vi "Calculate tf.vi"(7 "Open Interval? (T)":bool=TRUE, 11 "Waveform":T1) -> (3 "Tf Out":timestamp)   [LabVIEW 2020, in "WavBuf.lvclass"]
uses:
  WavBuf.lvclass
  Universal Controls/Waveform_Data.ctl
  <vilib>/Waveform/WDTOps.llb/WDT Get Final Time Value DBL.vi
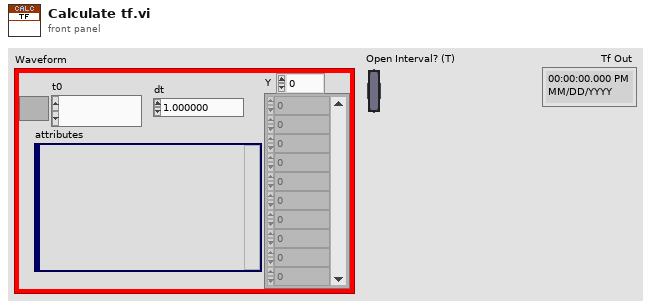
[diagram p1: front panel]
types:
  T1 = typedef "Waveform_Data.ctl" = waveform(dbl)
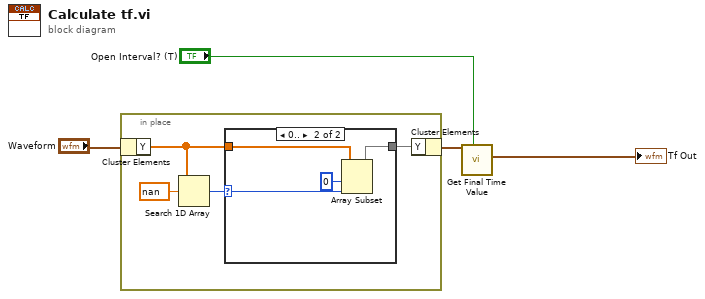
[diagram p0: block diagram]
diagram:
  n1 = in-place {
    n2 = in-place-cluster #1("Waveform") -> ("Y"=w6:dbl[])
    n3 = Search 1D Array(1D array=w6, element=nan) -> (index of element=w7:i32)  [unwired: 1 in]
    n4 = case shown="0.." w7 {
      selector: w7 -> [_ w10]
      tunnel: w6 -> [w9 w13]
      tunnel: [w9 w12] -> w5
      frame ..-1 {
      }
      frame 0.. {
        n5 = Array Subset(array=w13, index=0, length=w10) -> (w12:dbl[])
      }
    }
    n6 = in-place-cluster #1("Y"=w5) -> (w1:T1)
  }
  n7 = call-poly <vilib>:"Get Final Time Value.vi"("open interval? (T)"="Open Interval? (T)", "waveform in"=w1) -> ("tf"=→"Tf Out":timestamp)  [unwired: 7 in, 2 out]
